vi "pf Get Camera Property S.vi"(8 "error in (no error)":errorcluster, 9 "iSize":i32, 10 "pProperty":string, 11 "iPort":i32) -> (0 "error out":errorcluster, 2 "pValue out":string, 3 "function return":i32)   [LabVIEW 2012, in "Photonfocus_Toolkit.lvlib"]
doc: "PFCONFIG_API int pfGetCameraPropertyS(const char* pProperty, char* pValue, int iSize);"
uses:
  <userlib>/Photonfocus Toolkit/Photonfocus_Toolkit.lvlib
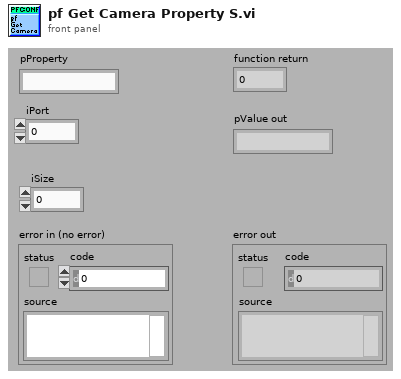
[diagram p1: front panel]
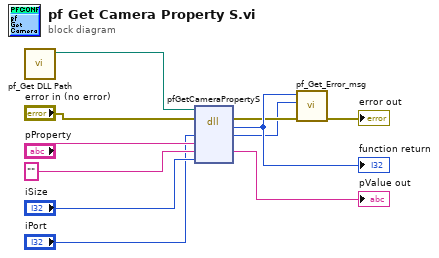
[diagram p0: block diagram]
diagram:
  n1 = call <userlib>:"pf_Get DLL Path.vi"() -> ("DLL path"=w3:path)  [unwired: 1 in, 10 out]
  n2 = dll-call lib="S:/Progetti/Photonfocus/Codice/DEV/PFConfig_lvlib/PFConfig.*" fn="pfGetCameraPropertyS"(path in=w3, error in="error in (no error)", "iPort"="iPort", "pProperty"="pProperty", "pValue"="", "iSize"="iSize") -> (error out=w5:errorcluster, "return type"=w11:i32, "iPort"=w1:i32, "pValue"=→"pValue out":string)  [unwired: 3 in, 1 out]
  "function return" <- w11
  n3 = call <userlib>:"pf_Get_Error_msg.vi"("error in (no error)"=w5, "iPort"=w1, "error code"=w11) -> ("error out"=→"error out":errorcluster)  [unwired: 8 out]
